vi "Display Info.vi"(7 "Layout ref":refnum<vi>, 8 "error in (no error)":errorcluster, 9 "Modify (F) /Add [T]":bool, 10 "Names in use":string[](array[string]), 11 "Pulseblaster in":refnum<class "Pulseblaster.lvclass">) -> (0 "error out":errorcluster, 1 "Names in use out":string[](array[string]), 2 "Changes Made?":bool, 3 "Pulseblaster out":refnum<class "Pulseblaster.lvclass">)   [LabVIEW 2013, in "Pulseblaster.lvclass"]
uses:
  Pulseblaster.lvclass
  TypeDefs/ColumnAppearCluster.ctl
  TypeDefs/DigitalColumnAppearCluster.ctl
  ColumnVIs/Column/Column.lvclass
  ColumnVIs/TriggerCol/TriggerCol.lvclass
  ColumnVIs/DigitalCol/DigitalCol.lvclass
  Globals/DisabledColorGlobal.vi
panel:
  out "Digital Cols":refnum<class "Column.lvclass">[](array[class])
  in  "Set All Digitals":T1={"Column Name"="", "Width"=18, "Bkgd"=[1985280, 6618880, 14090026], "Text"=[16448250, 0, 0]}
  in  "Trigger Line?":bool[](array[boolean])=[FALSE, FALSE, FALSE, FALSE, FALSE, FALSE, FALSE, FALSE, FALSE, FALSE, FALSE, FALSE, FALSE, FALSE, FALSE, FALSE, FALSE, FALSE, TRUE, TRUE, TRUE, TRUE, TRUE, TRUE]
  in  "Digital Columns":T1[](array[typedef])
  in  "Group Column":T1={"Column Name"="", "Width"=18, "Bkgd"=[1985280, 6618880, 14090026], "Text"=[16448250, 0, 0]}
  in  "Master Columns":T2[](array[typedef])
  in  "Cancel":bool
  in  "Done":bool
  in  "Device Description":string
  in  "Name":string
  # "Lines marked above will be disabled since they are programmed\nautomatically for triggering slave devices."
  # "0                          4                          8                         12                        16                        20"
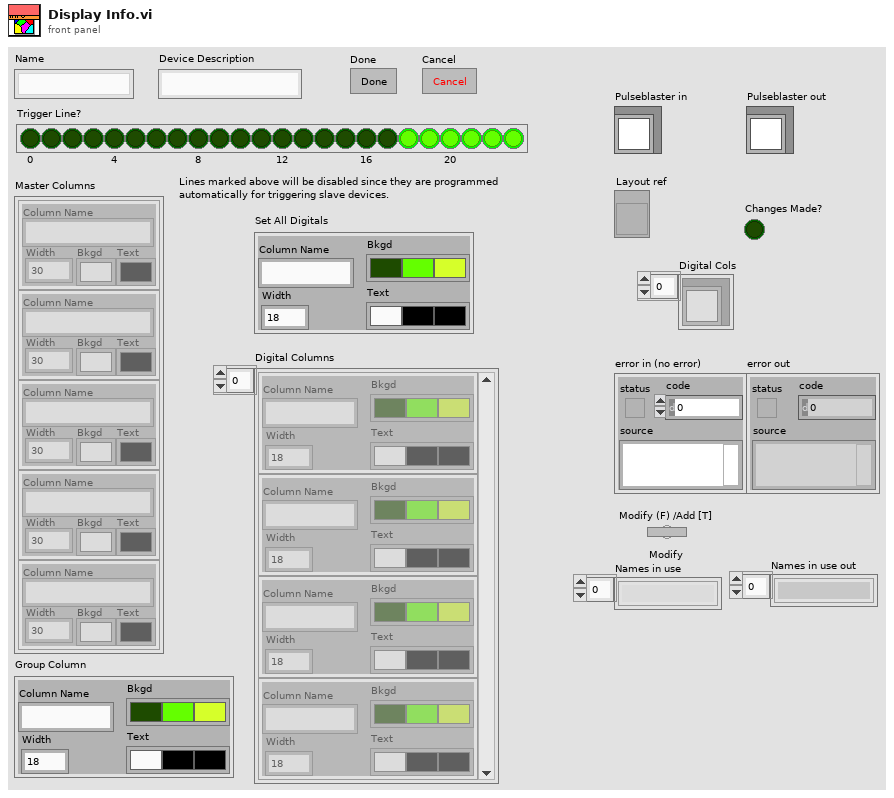
[diagram p1: front panel]
types:
  T1 = typedef "DigitalColumnAppearCluster.ctl" = cluster{"Column Name":string, "Width":u32, "Bkgd":u32[], "Text":u32[]}
  T2 = typedef "ColumnAppearCluster.ctl" = cluster{"Column Name":string, "Width":u32, "Bkgd":u32[], "Text":u32[]}
  T3 = cluster{"Column Name":bool, "Width":bool, "Bkgd":bool[], "Text":bool[]}[]
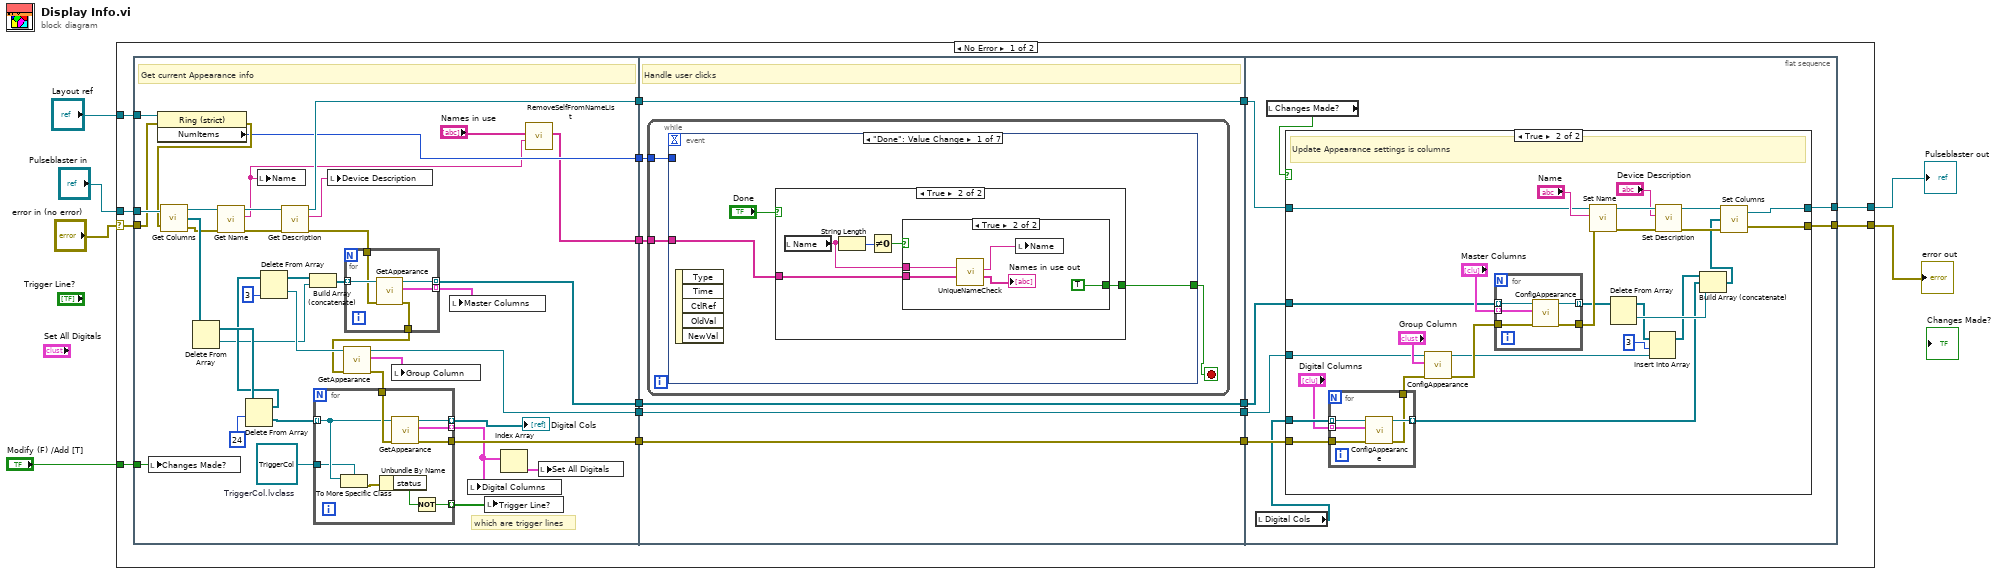
[diagram p0: block diagram]
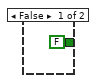
[diagram p2: hidden frame]
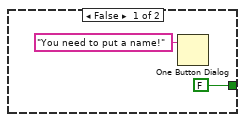
[diagram p3: hidden frame]
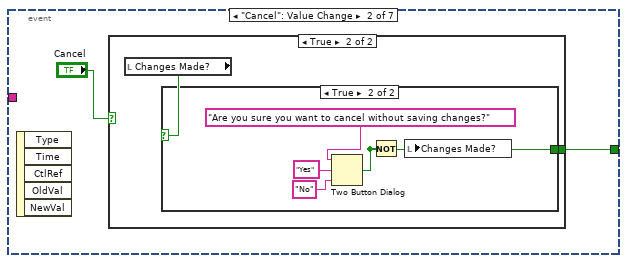
[diagram p4: hidden frame]
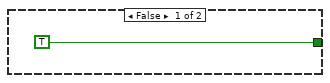
[diagram p6: hidden frame]
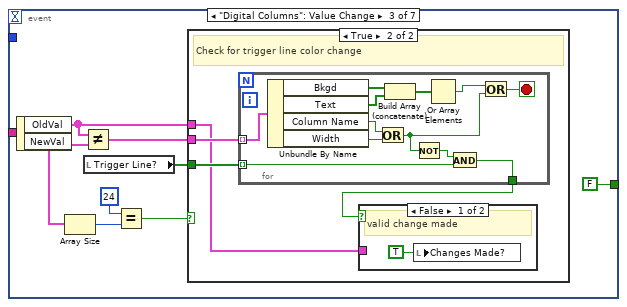
[diagram p7: hidden frame]
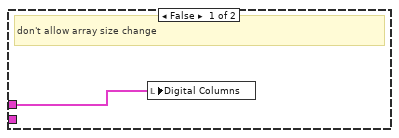
[diagram p8: hidden frame]
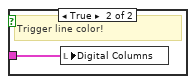
[diagram p9: hidden frame]
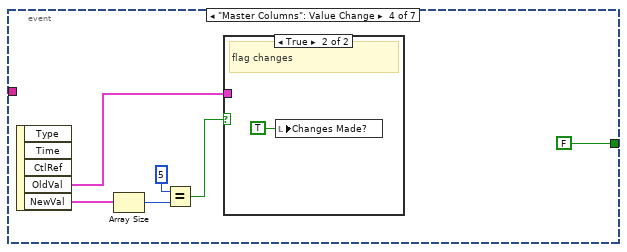
[diagram p10: hidden frame]
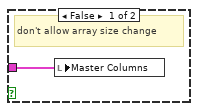
[diagram p11: hidden frame]
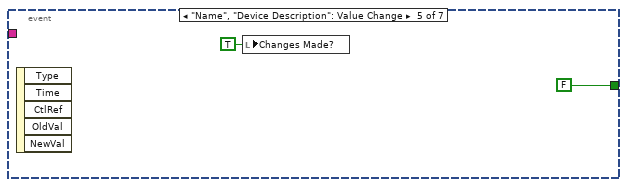
[diagram p12: hidden frame]
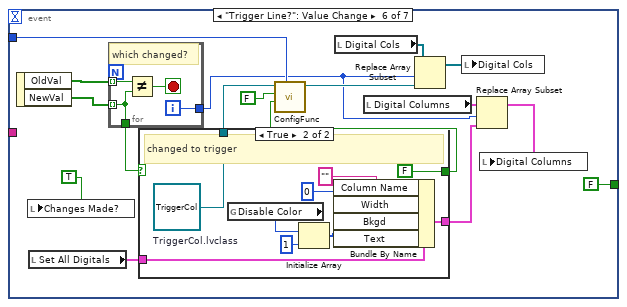
[diagram p13: hidden frame]
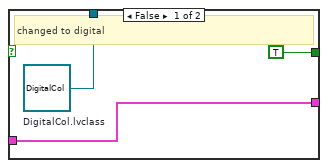
[diagram p14: hidden frame]
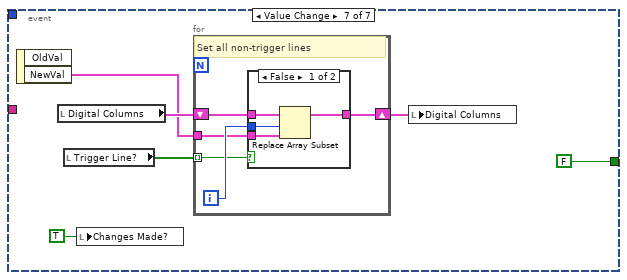
[diagram p15: hidden frame]
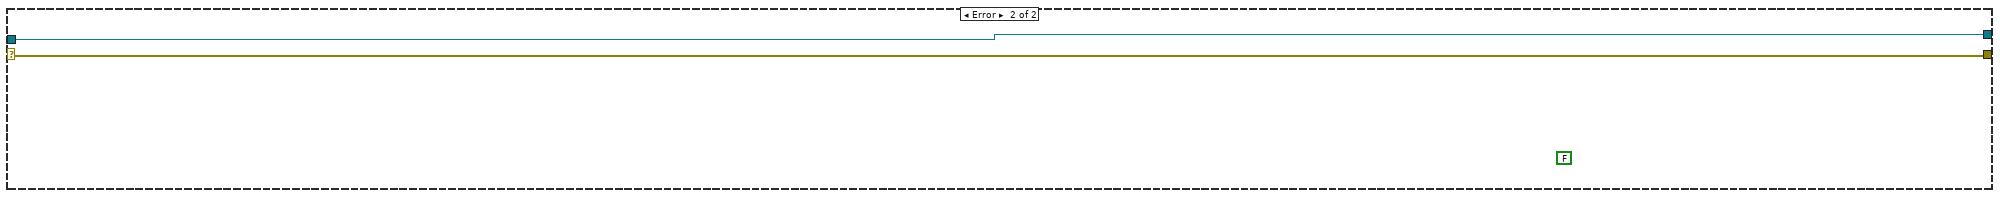
[diagram p18: hidden frame]
diagram:
  n1 = case shown="No Error" "error in (no error)" {
    selector: "error in (no error)" -> [w15 w244]
    tunnel: [w17 w245] -> w5
    tunnel: "Pulseblaster in" -> [w22 w245]
    tunnel: [w16 w244] -> w3
    tunnel: "Layout ref" -> [w10 _]
    tunnel: "Modify (F) /Add [T]" -> [w8 _]
    frame No Error {
      n2 = flat-sequence {
        tunnel: w22 -> [w49]
        tunnel: [w50] -> w21
        tunnel: [w39] -> w19
        tunnel: w15 -> [w29]
        tunnel: [w38] -> w14
        tunnel: [w37] -> w13
        tunnel: w10 -> [w30]
        tunnel: [w27] -> w9
        tunnel: w8 -> [w26]
        tunnel: [w23] -> w7
        tunnel: w21 -> [w80]
        tunnel: [w80] -> w20
        tunnel: w19 -> [w79]
        tunnel: [w79] -> w18
        tunnel: w14 -> [w78]
        tunnel: w13 -> [w77]
        tunnel: [w78] -> w12
        tunnel: [w77] -> w11
        tunnel: w9 -> [w76]
        tunnel: w7 -> [w75]
        tunnel: w20 -> [w203]
        tunnel: w18 -> [w199]
        tunnel: [w202] -> w17
        tunnel: [w201] -> w16
        tunnel: w12 -> [w200]
        tunnel: w11 -> [w198]
        frame #0 {
          w33 = refnum<class "TriggerCol.lvclass"> refnum  # TriggerCol.lvclass
          # "which are trigger lines"
          # "Get current Appearance info"
          n3 = local write "Changes Made?"(w26) -> ()
          n4 = property class="Ring (strict)"(reference=w30, error in=w29) -> (error out=w28:errorcluster, "NumItems"=w27:u32)  [unwired: 1 out]
          n5 = call-dynamic "Get Columns.vi"("Device in"=w49, "error in (no error)"=w28) -> ("Device out"=w47:refnum<class "Pulseblaster.lvclass">, "Columns"=w58:refnum<class "Column.lvclass">[], "error out"=w46:errorcluster)
          n6 = Delete From Array(array=w58) -> (deleted portion=w36:refnum<class "Column.lvclass">, array with subset deleted=w57:refnum<class "Column.lvclass">[])  [unwired: 2 in]
          n7 = call-dynamic "Get Name.vi"("error in (no error)"=w46, "Device in"=w47) -> ("error out"=w48:errorcluster, "Name"=w24:string, "Device out"=w60:refnum<class "Pulseblaster.lvclass">)  [unwired: 7 in]
          n8 = Delete From Array(array=w57, length=24) -> (deleted portion=w45:refnum<class "Column.lvclass">[], array with subset deleted=w44:refnum<class "Column.lvclass">[])  [unwired: 1 in]
          n9 = local write "Name"(w24) -> ()
          n10 = Delete From Array(array=w44, index=3) -> (deleted portion=w43:refnum<class "Column.lvclass">, array with subset deleted=w52:refnum<class "Column.lvclass">[])  [unwired: 1 in]
          n11 = call-dynamic "Get Description.vi"("error in (no error)"=w48, "Device in"=w60) -> ("error out"=w40:errorcluster, "Device Description"=w59:string, "Device out"=w50:refnum<class "Pulseblaster.lvclass">)  [unwired: 7 in]
          n12 = Build Array (concatenate)(w52, w36) -> (w51:refnum<class "Column.lvclass">[])
          n13 = local write "Device Description"(w59) -> ()
          n14 = for {
            tunnel: w51 -> [w74] mode=indexing
            tunnel: [w73] -> w55 mode=indexing
            tunnel: w40 -> [w72]
            tunnel: [w71] -> w41
            tunnel: [w70] -> w38 mode=indexing
            n15 = call "GetAppearance.vi"("error in (no error)"=w72, "Column in"=w74) -> ("error out"=w71:errorcluster, "Column Appearance"=w73:T2, "Column out"=w70:refnum<class "Column.lvclass">)  [unwired: 7 in]
          }
          n16 = call "GetAppearance.vi"("error in (no error)"=w41, "Column in"=w43) -> ("error out"=w42:errorcluster, "Column Appearance"=w54:T2, "Column out"=w37:refnum<class "Column.lvclass">)  [unwired: 7 in]
          n17 = for {
            tunnel: w45 -> [w65] mode=indexing
            tunnel: [w69] -> w35 mode=indexing
            tunnel: [w68] -> w39
            tunnel: w42 -> [w67]
            tunnel: [w66] -> w31 mode=indexing
            tunnel: w33 -> [w64]
            tunnel: [w62] -> w32 mode=indexing
            n18 = To More Specific Class(target class=w64, reference=w65) -> (error out=w63:errorcluster)  [unwired: 1 in, 1 out]
            n19 = Unbundle By Name(w63) -> ("status"=w61:bool)
            n20 = call "GetAppearance.vi"("error in (no error)"=w67, "Column in"=w65) -> ("error out"=w68:errorcluster, "Column Appearance"=w69:T2, "Column out"=w66:refnum<class "Column.lvclass">)  [unwired: 7 in]
            n21 = Not(x=w61) -> (.not. x?=w62:bool)
          }
          "Digital Cols" <- w31
          n22 = local write "Group Column"(w54) -> ()
          n23 = local write "Master Columns"(w55) -> ()
          n24 = local write "Digital Columns"(w35) -> ()
          n25 = local write "Trigger Line?"(w32) -> ()
          n26 = Index Array(array=w35) -> (element=w34:T2)  [unwired: 1 in]
          n27 = call "RemoveSelfFromNameList.vi"("self Name"=w24, "Names in use"="Names in use") -> ("Reserved Names"=w23:string[])  [unwired: 9 in]
          n28 = local write "Set All Digitals"(w34) -> ()
        }
        frame #1 {
          # "Handle user clicks"
          n29 = while {
            tunnel: w76 -> [w82]
            tunnel: w75 -> [w81]
            stop <- w83 stop-if-true
            n30 = event shown="[0] \"Done\": Value Change" {
              selector: _ -> [_ _ _ _ _ _ _]
              dyn-events: _ -> [_ _ _ _ _ _ _]
              timeout: _ -> [_ _ _ _ _ _ _]
              tunnel: [w85 w101 FALSE ("T button?") FALSE ("T button?") FALSE ("T button?") FALSE ("T button?") FALSE ("T button?")] -> w83
              tunnel: w82 -> [_ _ _ _ _ w155 _]
              tunnel: w81 -> [w84 _ _ _ _ _ _]
              event "Done": Value Change {
                n31 = event-data() -> ()  [unwired: 1 in, 5 out]
                n32 = case shown="True" "Done" {
                  tunnel: [FALSE w90] -> w85
                  tunnel: w84 -> [_ w88]
                  frame False {
                  }
                  frame True {
                    n33 = local read "Name"() -> (w89:string)
                    n34 = String Length(string=w89) -> (length=w92:i32)
                    n35 = Not Equal To 0?(x=w92) -> (x != 0?=w91:bool)
                    n36 = case shown="True" w91 {
                      tunnel: [FALSE TRUE] -> w90
                      tunnel: w89 -> [_ w98]
                      tunnel: w88 -> [_ w96]
                      frame False {
                        n37 = One Button Dialog(message="You need to put a name!") -> ()  [unwired: 1 in, 1 out]
                      }
                      frame True {
                        n38 = call "UniqueNameCheck.vi"("Names in use"=w96, "Device Name"=w98) -> ("Names in use out"=→"Names in use out":string[], "Unique name"=w97:string)  [unwired: 8 in]
                        n39 = local write "Name"(w97) -> ()
                      }
                    }
                  }
                }
              }
              event "Cancel": Value Change {
                n40 = event-data() -> ()  [unwired: 1 in, 5 out]
                n41 = case shown="True" "Cancel" {
                  selector: "Cancel" -> [w102 _]
                  tunnel: [w102 w104] -> w101
                  frame False {
                  }
                  frame True {
                    n42 = local read "Changes Made?"() -> (w103:bool)
                    n43 = case shown="True" w103 {
                      tunnel: [TRUE w107] -> w104
                      frame False {
                      }
                      frame True {
                        n44 = Two Button Dialog(message="Are you sure you want to cancel without saving changes?", 1:"No", 2:"Yes") -> (T button?=w107:bool)
                        n45 = Not(x=w107) -> (.not. x?=w106:bool)
                        n46 = local write "Changes Made?"(w106) -> ()
                      }
                    }
                  }
                }
              }
              event "Digital Columns": Value Change {
                n47 = event-data() -> ("OldVal"=w111:T1[], "NewVal"=w113:T1[])  [unwired: 1 in]
                n48 = Array Size(array=w113) -> (size(s)=w117:i32)
                n49 = Not Equal?(x=w111, y=w113) -> (x != y?=w112:T3)
                n50 = local read "Trigger Line?"() -> (w114:bool[])
                n51 = Equal?(x=24 ("y"), y=w117) -> (x = y?=w118:bool)
                n52 = case shown="True" w118 {
                  tunnel: w111 -> [w119 w120]
                  tunnel: w114 -> [_ w122]
                  tunnel: w112 -> [_ w123]
                  frame False {
                    # "don't allow array size change"
                    n53 = local write "Digital Columns"(w119) -> ()
                  }
                  frame True {
                    # "Check for trigger line color change"
                    n54 = for {
                      tunnel: w123 -> [w137] mode=indexing
                      tunnel: w122 -> [w129] mode=indexing
                      tunnel: [w128] -> w121
                      stop <- w133 stop-if-true
                      n55 = Unbundle By Name(w137) -> ("Bkgd"=w136:bool[], "Text"=w135:bool[], "Column Name"=w131:bool, "Width"=w130:bool)
                      n56 = Or(x=w131, y=w130) -> (x .or. y?=w127:bool)
                      n57 = Build Array (concatenate)(w136, w135) -> (w134:bool[])
                      n58 = Not(x=w127) -> (.not. x?=w126:bool)
                      n59 = Or Array Elements(Boolean array=w134) -> (logical OR=w132:bool)
                      n60 = And(x=w126, y=w129) -> (x .and. y?=w128:bool)
                      n61 = Or(x=w132, y=w127) -> (x .or. y?=w133:bool)
                    }
                    n62 = case shown="False" w121 {
                      tunnel: w120 -> [_ w125]
                      frame False {
                        # "valid change made"
                        n63 = local write "Changes Made?"(TRUE ("Changes Made?")) -> ()
                      }
                      frame True {
                        # "Trigger line color!"
                        n64 = local write "Digital Columns"(w125) -> ()
                      }
                    }
                  }
                }
              }
              event "Master Columns": Value Change {
                n65 = event-data() -> ("OldVal"=w141:T2[], "NewVal"=w143:T2[])  [unwired: 1 in, 3 out]
                n66 = Array Size(array=w143) -> (size(s)=w140:i32)
                n67 = Equal?(x=5 ("y"), y=w140) -> (x = y?=w142:bool)
                n68 = case shown="True" w142 {
                  tunnel: w141 -> [w144 _]
                  frame False {
                    # "don't allow array size change"
                    n69 = local write "Master Columns"(w144) -> ()
                  }
                  frame True {
                    # "flag changes"
                    n70 = local write "Changes Made?"(TRUE ("Changes Made?")) -> ()
                  }
                }
              }
              event "Name", "Device Description": Value Change {
                n71 = event-data() -> ()  [unwired: 1 in, 5 out]
                n72 = local write "Changes Made?"(TRUE) -> ()
              }
              event "Trigger Line?": Value Change {
                n73 = event-data() -> ("OldVal"=w164:bool[], "NewVal"=w163:bool[])  [unwired: 1 in]
                n74 = local write "Changes Made?"(TRUE) -> ()
                n75 = local read "Set All Digitals"() -> (w161:T1)
                n76 = for {
                  tunnel: w164 -> [w180] mode=indexing
                  tunnel: w163 -> [w178] mode=indexing
                  tunnel: [w178] -> w162
                  tunnel: [w177] -> w149
                  i -> [w177]
                  stop <- w179 stop-if-true
                  # "which changed?"
                  n77 = Not Equal?(x=w180, y=w178) -> (x != y?=w179:bool)
                }
                n78 = case shown="True" w162 {
                  tunnel: w161 -> [w166 w172]
                  tunnel: [TRUE ("isVariable?") FALSE ("isVariable?")] -> w157
                  tunnel: [w166 w170] -> w148
                  tunnel: [w165 w169] -> w156
                  frame False {
                    w165 = refnum<class "DigitalCol.lvclass"> refnum  # DigitalCol.lvclass
                    # "changed to digital"
                  }
                  frame True {
                    w169 = refnum<class "TriggerCol.lvclass"> refnum  # TriggerCol.lvclass
                    # "changed to trigger"
                    n79 = global read "DisabledColorGlobal.vi" "Disable Color"() -> (w173:u32)
                    n80 = Initialize Array(w173, 1 ("dimension size")) -> (w175:u32[])
                    n81 = Bundle By Name(cluster=w172, "Column Name"="", "Width"=u32 0 ("Width (60)"), "Bkgd"=w175, "Text"=w175) -> (w170:T1)
                  }
                }
                n82 = call "ConfigFunc.vi"("Num Layouts (ignored)"=w155, "isVariable? (True)"=w157, "Disableable? (True)"=FALSE, "Column in"=w156) -> ("Column out"=w152:refnum<class "Column.lvclass">)  [unwired: 6 in, 1 out]
                n83 = local read "Digital Cols"() -> (w160:refnum<class "Column.lvclass">[])
                n84 = local read "Digital Columns"() -> (w151:T1[])
                n85 = Replace Array Subset(array=w160, new element=w152, index=w149) -> (w159:refnum<class "Column.lvclass">[])
                n86 = local write "Digital Cols"(w159) -> ()
                n87 = Replace Array Subset(array=w151, new element=w148, index=w149) -> (w150:T1[])
                n88 = local write "Digital Columns"(w150) -> ()
              }
              event Value Change {
                n89 = event-data() -> ("NewVal"=w184:T1)  [unwired: 1 in, 1 out]
                n90 = local read "Digital Columns"() -> (w186:T1[])
                n91 = local read "Trigger Line?"() -> (w185:bool[])
                n92 = local write "Changes Made?"(TRUE) -> ()
                n93 = for {
                  tunnel: w185 -> [w188] mode=indexing
                  tunnel: w184 -> [w189]
                  shift-right: [w187] -> w183
                  shift-left: w186 -> [w191]
                  i -> [w190]
                  # "Set all non-trigger lines"
                  n94 = case shown="False" w188 {
                    tunnel: w191 -> [w195 w196]
                    tunnel: w190 -> [w194 _]
                    tunnel: w189 -> [w193 _]
                    tunnel: [w192 w196] -> w187
                    frame False {
                      n95 = Replace Array Subset(array=w195, new element=w193, index=w194) -> (w192:T1[])
                    }
                    frame True {
                    }
                  }
                }
                n96 = local write "Digital Columns"(w183) -> ()
              }
            }
          }
        }
        frame #2 {
          n97 = local read "Digital Cols"() -> (w197:refnum<class "Column.lvclass">[])
          n98 = local read "Changes Made?"() -> (w204:bool)
          n99 = case shown="True" w204 {
            tunnel: w203 -> [w206 w223]
            tunnel: [w205 w225] -> w201
            tunnel: [w206 w224] -> w202
            tunnel: w200 -> [_ w222]
            tunnel: w199 -> [w205 w221]
            tunnel: w197 -> [_ w220]
            tunnel: w198 -> [_ w216]
            frame False {
            }
            frame True {
              # "Update Appearance settings is columns"
              n100 = for {
                tunnel: "Digital Columns" -> [w238] mode=indexing
                tunnel: [w237] -> w207 mode=indexing
                tunnel: [w236] -> w218
                tunnel: w220 -> [w235] mode=indexing
                tunnel: w221 -> [w234]
                n101 = call "ConfigAppearance.vi"("error in (no error)"=w234, "Column Appearance"=w238, "Column in"=w235) -> ("error out"=w236:errorcluster, "Column out"=w237:refnum<class "Column.lvclass">)  [unwired: 7 in]
              }
              n102 = call "ConfigAppearance.vi"("error in (no error)"=w218, "Column Appearance"="Group Column", "Column in"=w216) -> ("error out"=w217:errorcluster, "Column out"=w210:refnum<class "Column.lvclass">)  [unwired: 7 in]
              n103 = for {
                tunnel: "Master Columns" -> [w243] mode=indexing
                tunnel: [w242] -> w212 mode=indexing
                tunnel: [w241] -> w214
                tunnel: w222 -> [w240] mode=indexing
                tunnel: w217 -> [w239]
                n104 = call "ConfigAppearance.vi"("error in (no error)"=w239, "Column Appearance"=w243, "Column in"=w240) -> ("error out"=w241:errorcluster, "Column out"=w242:refnum<class "Column.lvclass">)  [unwired: 7 in]
              }
              n105 = call-dynamic "Set Name.vi"("error in (no error)"=w214, "Name"="Name", "Device in"=w223) -> ("error out"=w233:errorcluster, "Device out"=w232:refnum<class "Pulseblaster.lvclass">)  [unwired: 7 in]
              n106 = Delete From Array(array=w212) -> (deleted portion=w211:refnum<class "Column.lvclass">, array with subset deleted=w209:refnum<class "Column.lvclass">[])  [unwired: 2 in]
              n107 = Insert Into Array(array=w209, index=3, new element=w210) -> (w208:refnum<class "Column.lvclass">[])
              n108 = call-dynamic "Set Description.vi"("error in (no error)"=w233, "Device Description"="Device Description", "Device in"=w232) -> ("error out"=w215:errorcluster, "Device out"=w231:refnum<class "Pulseblaster.lvclass">)  [unwired: 7 in]
              n109 = Build Array (concatenate)(w208, w207, w211) -> (w213:refnum<class "Column.lvclass">[])
              n110 = call-dynamic "Set Columns.vi"("error in (no error)"=w215, "Columns in"=w213, "Pulseblaster in"=w231) -> ("error out"=w225:errorcluster, "Pulseblaster out"=w224:refnum<class "Pulseblaster.lvclass">)  [unwired: 1 in]
            }
          }
        }
      }
    }
    frame Error {
      (unwired) FALSE
    }
  }
  "error out" <- w3
  "Pulseblaster out" <- w5
